vi "Compare_Global_Values_Modify_Cost_f()-2.vi"(4 "[IN] Lengths":u8[](array[numeric]), 5 "error IN":errorcluster, 6 "[IN] Linearity":u8[](array[numeric]), 7 "[IN] Array of Mean\n(dR) - Problem dR":dbl[](array[numeric]), 8 "[IN] SD(Areas)":dbl[](array[numeric]), 9 "[IN] Array of Mean(Areas)\n - Problem finish Area":dbl[](array[numeric]), 10 "[IN] SD(dR)":dbl[](array[numeric]), 11 "[IN] Cost function":i8[](array[numeric])) -> (0 "error OUT":errorcluster, 3 "[OUT] Cost function":i8[](array[numeric]))   [LabVIEW 2013]
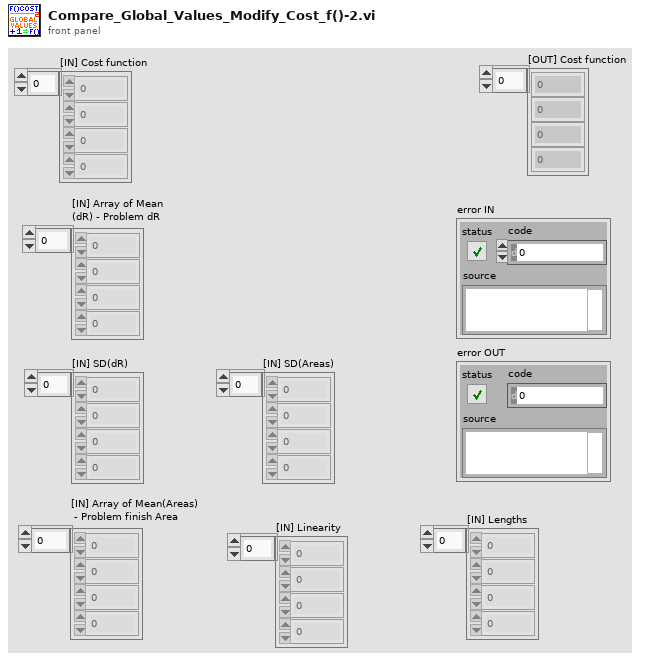
[diagram p1: front panel]
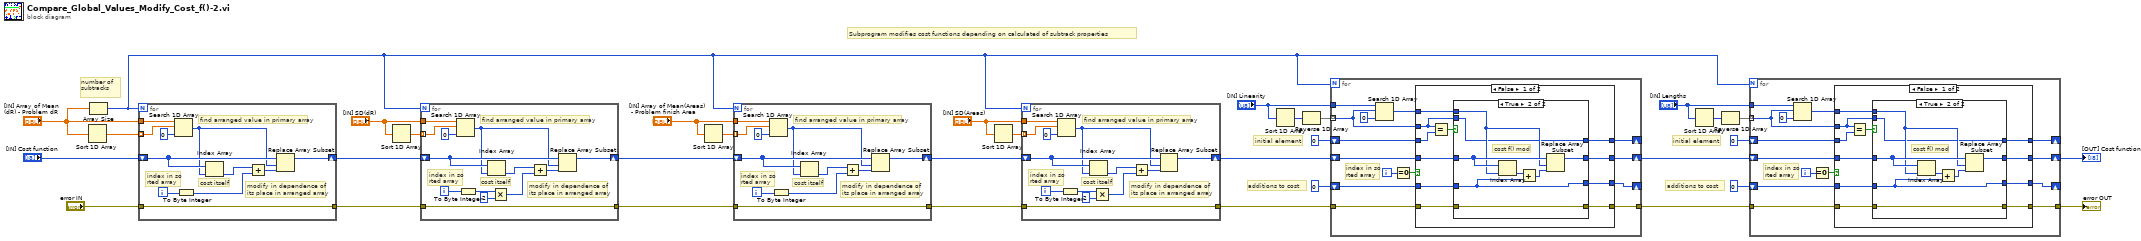
[diagram p0: block diagram]
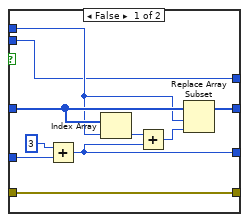
[diagram p2: hidden frame]
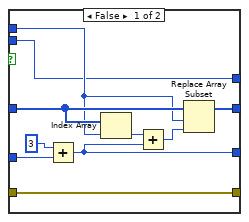
[diagram p4: hidden frame]
diagram:
  # "additions to cost"
  # "initial element"
  # "additions to cost"
  # "initial element"
  # "Subprogram modifies cost functions depending on calculated of subtrack properties"
  # "number of \nsubtracks"
  n1 = Sort 1D Array(array="[IN] Array of Mean\n(dR) - Problem dR") -> (sorted array=w33:dbl[])
  n2 = Array Size(array="[IN] Array of Mean\n(dR) - Problem dR") -> (size(s)=w1:i32)
  n3 = for {
    N: w1 -> [_]
    tunnel: w33 -> [w42] mode=indexing
    tunnel: "[IN] Array of Mean\n(dR) - Problem dR" -> [w44]
    shift-right: [w35] -> w30
    shift-left: "[IN] Cost function" -> [w41]
    tunnel: "error IN" -> [w34]
    tunnel: [w34] -> w24
    i -> [w37]
    # "modify in dependence of \nits place in arranged array"
    # "find arranged value in primary array"
    # "index in so\nrted array"
    # "cost itself"
    n4 = Search 1D Array(1D array=w44, element=w42, start index (0)=0) -> (index of element=w40:i32)
    n5 = To Byte Integer(number=w37) -> (8bit integer=w36:i8)
    n6 = Index Array(array=w41, index=w40) -> (element=w39:i8)
    n7 = Add(x=w39, y=w36) -> (x+y=w38:i8)
    n8 = Replace Array Subset(array=w41, new element=w38, index=w40) -> (w35:i8[])
  }
  n9 = Sort 1D Array(array="[IN] SD(dR)") -> (sorted array=w28:dbl[])
  n10 = for {
    N: w1 -> [_]
    tunnel: w28 -> [w55] mode=indexing
    tunnel: "[IN] SD(dR)" -> [w57]
    shift-right: [w49] -> w26
    shift-left: w30 -> [w54]
    tunnel: w24 -> [w48]
    tunnel: [w48] -> w23
    i -> [w50]
    # "modify in dependence of \nits place in arranged array"
    # "find arranged value in primary array"
    # "index in so\nrted array"
    # "cost itself"
    n11 = Search 1D Array(1D array=w57, element=w55, start index (0)=0) -> (index of element=w53:i32)
    n12 = To Byte Integer(number=w50) -> (8bit integer=w47:i8)
    n13 = Index Array(array=w54, index=w53) -> (element=w52:i8)
    n14 = Multiply(x=w47, y=i8 2) -> (x*y=w45:i8)
    n15 = Add(x=w52, y=w45) -> (x+y=w51:i8)
    n16 = Replace Array Subset(array=w54, new element=w51, index=w53) -> (w49:i8[])
  }
  n17 = Sort 1D Array(array="[IN] Array of Mean(Areas)\n - Problem finish Area") -> (sorted array=w27:dbl[])
  n18 = for {
    N: w1 -> [_]
    tunnel: w27 -> [w66] mode=indexing
    tunnel: "[IN] Array of Mean(Areas)\n - Problem finish Area" -> [w68]
    shift-right: [w59] -> w19
    shift-left: w26 -> [w65]
    tunnel: w23 -> [w58]
    tunnel: [w58] -> w18
    i -> [w61]
    # "modify in dependence of \nits place in arranged array"
    # "find arranged value in primary array"
    # "index in so\nrted array"
    # "cost itself"
    n19 = Search 1D Array(1D array=w68, element=w66, start index (0)=0) -> (index of element=w64:i32)
    n20 = To Byte Integer(number=w61) -> (8bit integer=w60:i8)
    n21 = Index Array(array=w65, index=w64) -> (element=w63:i8)
    n22 = Add(x=w63, y=w60) -> (x+y=w62:i8)
    n23 = Replace Array Subset(array=w65, new element=w62, index=w64) -> (w59:i8[])
  }
  n24 = Sort 1D Array(array="[IN] SD(Areas)") -> (sorted array=w20:dbl[])
  n25 = for {
    N: w1 -> [_]
    tunnel: w20 -> [w79] mode=indexing
    tunnel: "[IN] SD(Areas)" -> [w81]
    shift-right: [w73] -> w13
    shift-left: w19 -> [w78]
    tunnel: w18 -> [w72]
    tunnel: [w72] -> w11
    i -> [w74]
    # "modify in dependence of \nits place in arranged array"
    # "find arranged value in primary array"
    # "index in so\nrted array"
    # "cost itself"
    n26 = Search 1D Array(1D array=w81, element=w79, start index (0)=0) -> (index of element=w77:i32)
    n27 = To Byte Integer(number=w74) -> (8bit integer=w71:i8)
    n28 = Index Array(array=w78, index=w77) -> (element=w76:i8)
    n29 = Multiply(x=w71, y=i8 2) -> (x*y=w69:i8)
    n30 = Add(x=w76, y=w69) -> (x+y=w75:i8)
    n31 = Replace Array Subset(array=w78, new element=w75, index=w77) -> (w73:i8[])
  }
  n32 = Sort 1D Array(array="[IN] Linearity") -> (sorted array=w16:u8[])
  n33 = Reverse 1D Array(array=w16) -> (reversed array=w15:u8[])
  n34 = for {
    N: w1 -> [_]
    tunnel: w15 -> [w91] mode=indexing
    tunnel: "[IN] Linearity" -> [w95]
    shift-right: [w89] -> w6
    shift-left: w13 -> [w90]
    shift-right: [w88] -> _
    shift-left: u8 0 -> [w87]
    shift-right: [w85] -> _
    shift-left: i8 0 -> [w86]
    tunnel: w11 -> [w83]
    tunnel: [w82] -> w5
    i -> [w93]
    # "index in so\nrted array"
    n35 = Search 1D Array(1D array=w95, element=w91, start index (0)=0) -> (index of element=w84:i32)
    n36 = Equal To 0?(x=w93) -> (x = 0?=w92:bool)
    n37 = case shown="False" w92 {
      tunnel: w91 -> [w101 w127]
      tunnel: [w100 w128] -> w89
      tunnel: w90 -> [w104 w128]
      tunnel: [w99 w127] -> w88
      tunnel: w87 -> [w106 _]
      tunnel: [w98 w126] -> w85
      tunnel: w86 -> [w102 w126]
      tunnel: w84 -> [w103 _]
      tunnel: w83 -> [w97 w125]
      tunnel: [w96 w125] -> w82
      frame False {
        n38 = Equal?(x=w101, y=w106) -> (x = y?=w105:bool)
        n39 = case shown="True" w105 {
          tunnel: w104 -> [w114 w122]
          tunnel: w103 -> [w111 w119]
          tunnel: w102 -> [w116 w121]
          tunnel: w101 -> [w109 w118]
          tunnel: [w110 w120] -> w100
          tunnel: [w109 w118] -> w99
          tunnel: [w108 w121] -> w98
          tunnel: w97 -> [w107 w117]
          tunnel: [w107 w117] -> w96
          frame False {
            n40 = Add(x=i8 3 ("y"), y=w116) -> (x+y=w108:i8)
            n41 = Index Array(array=w114, index=w111) -> (element=w113:i8)
            n42 = Add(x=w113, y=w108) -> (x+y=w112:i8)
            n43 = Replace Array Subset(array=w114, new element=w112, index=w111) -> (w110:i8[])
          }
          frame True {
            # "cost f() mod"
            n44 = Index Array(array=w122, index=w119) -> (element=w123:i8)
            n45 = Add(x=w123, y=w121) -> (x+y=w124:i8)
            n46 = Replace Array Subset(array=w122, new element=w124, index=w119) -> (w120:i8[])
          }
        }
      }
      frame True {
      }
    }
  }
  n47 = Sort 1D Array(array="[IN] Lengths") -> (sorted array=w10:u8[])
  n48 = Reverse 1D Array(array=w10) -> (reversed array=w9:u8[])
  n49 = for {
    N: w1 -> [_]
    tunnel: w9 -> [w138] mode=indexing
    tunnel: "[IN] Lengths" -> [w142]
    shift-right: [w136] -> w3
    shift-left: w6 -> [w137]
    shift-right: [w135] -> _
    shift-left: u8 0 -> [w134]
    shift-right: [w132] -> _
    shift-left: i8 0 -> [w133]
    tunnel: w5 -> [w130]
    tunnel: [w129] -> w2
    i -> [w140]
    # "index in so\nrted array"
    n50 = Search 1D Array(1D array=w142, element=w138, start index (0)=0) -> (index of element=w131:i32)
    n51 = Equal To 0?(x=w140) -> (x = 0?=w139:bool)
    n52 = case shown="False" w139 {
      tunnel: w138 -> [w148 w174]
      tunnel: [w147 w175] -> w136
      tunnel: w137 -> [w151 w175]
      tunnel: [w146 w174] -> w135
      tunnel: w134 -> [w153 _]
      tunnel: [w145 w173] -> w132
      tunnel: w133 -> [w149 w173]
      tunnel: w131 -> [w150 _]
      tunnel: w130 -> [w144 w172]
      tunnel: [w143 w172] -> w129
      frame False {
        n53 = Equal?(x=w148, y=w153) -> (x = y?=w152:bool)
        n54 = case shown="True" w152 {
          tunnel: w151 -> [w161 w169]
          tunnel: w150 -> [w158 w166]
          tunnel: w149 -> [w163 w168]
          tunnel: w148 -> [w156 w165]
          tunnel: [w157 w167] -> w147
          tunnel: [w156 w165] -> w146
          tunnel: [w155 w168] -> w145
          tunnel: w144 -> [w154 w164]
          tunnel: [w154 w164] -> w143
          frame False {
            n55 = Add(x=i8 3 ("y"), y=w163) -> (x+y=w155:i8)
            n56 = Index Array(array=w161, index=w158) -> (element=w160:i8)
            n57 = Add(x=w160, y=w155) -> (x+y=w159:i8)
            n58 = Replace Array Subset(array=w161, new element=w159, index=w158) -> (w157:i8[])
          }
          frame True {
            # "cost f() mod"
            n59 = Index Array(array=w169, index=w166) -> (element=w170:i8)
            n60 = Add(x=w170, y=w168) -> (x+y=w171:i8)
            n61 = Replace Array Subset(array=w169, new element=w171, index=w166) -> (w167:i8[])
          }
        }
      }
      frame True {
      }
    }
  }
  "[OUT] Cost function" <- w3
  "error OUT" <- w2
